vi "Drive Helper.vi"(1 "QuickTurn":bool, 2 "AutoShift":bool, 3 "Wheel Speed":dbl, 5 "Throttle":dbl(slide) scale=-1.0..1.0, 9 "Turn":dbl(slide) scale=-1.0..1.0, 12 "ForceHigh":bool, 13 "ForceLow":bool) -> (6 "Left Output":dbl(slide) scale=-1.0..1.0, 8 "isHighGear":bool, 10 "Right Output":dbl(slide) scale=-1.0..1.0)   [LabVIEW 2014]
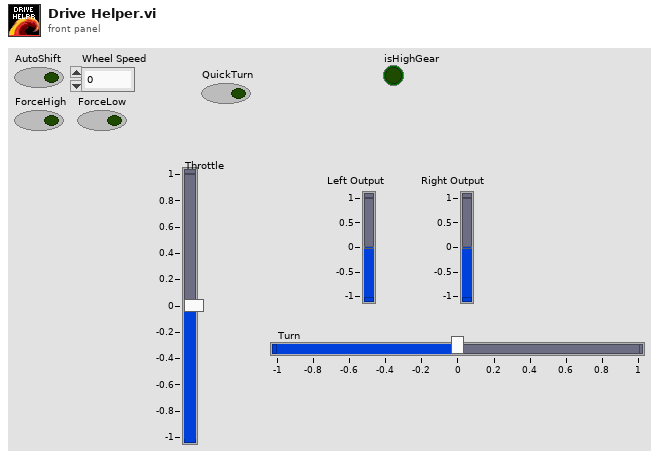
[diagram p1: front panel]
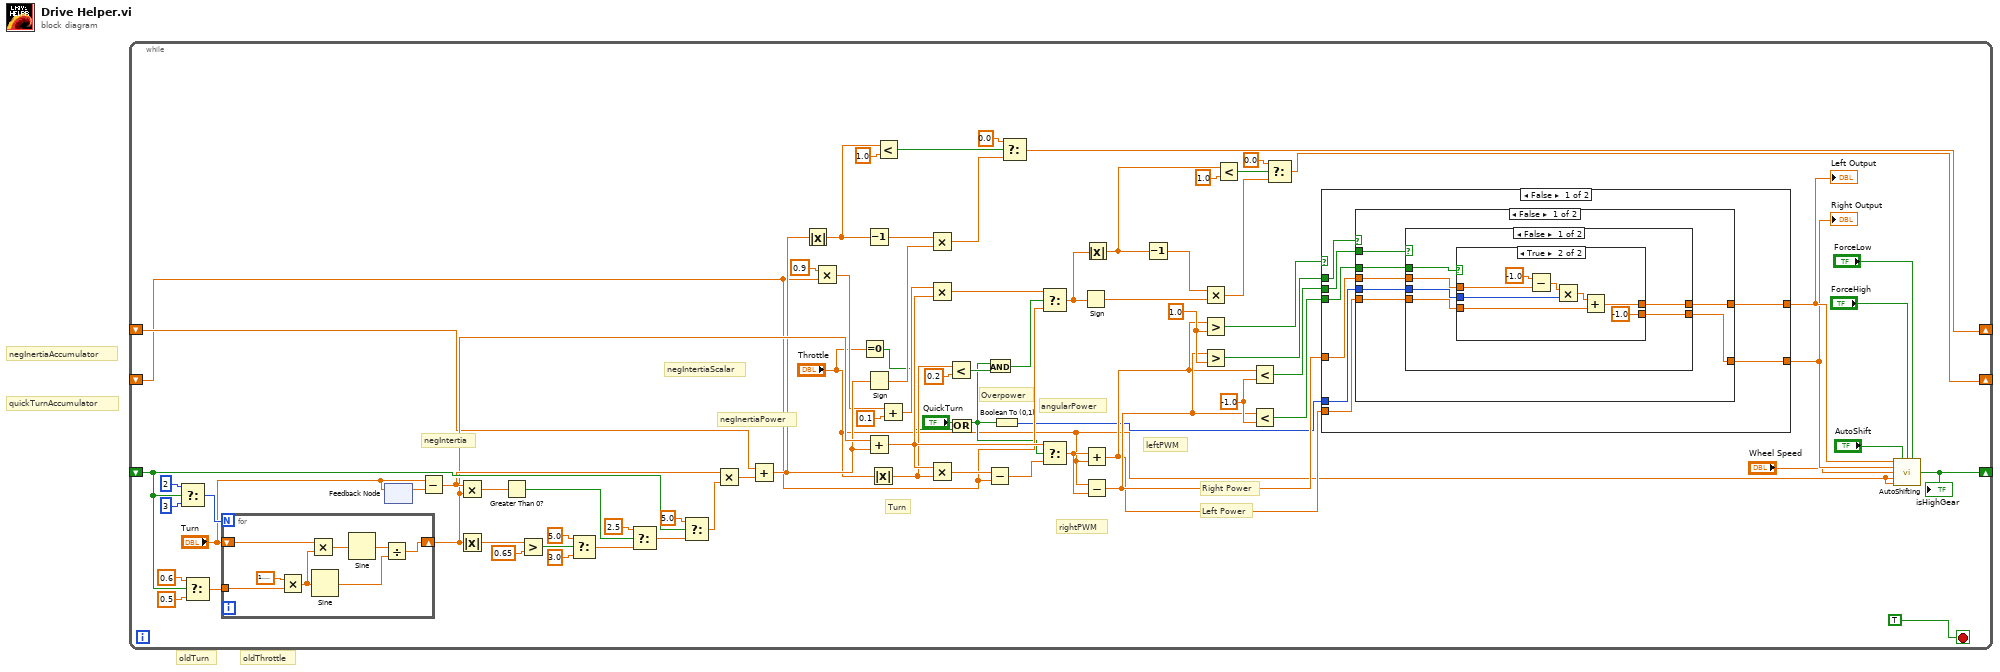
[diagram p0: block diagram]
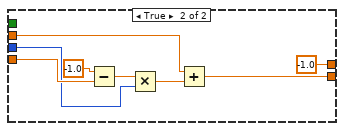
[diagram p3: hidden frame]
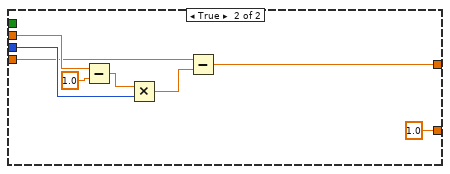
[diagram p4: hidden frame]
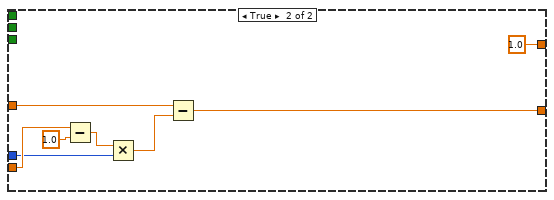
[diagram p5: hidden frame]
diagram:
  # "quickTurnAccumulator"
  # "negInertiaAccumulator"
  # "oldThrottle"
  # "oldTurn"
  n1 = while {
    shift-right: [w77] -> _
    shift-left: _ -> [w69]
    shift-right: [w45] -> _
    shift-left: _ -> [w42]
    shift-right: [w21] -> _
    shift-left: _ -> [w31]
    stop <- TRUE ("Stop") stop-if-true
    w17 = -1.0 ("y")
    w14 = 1.0 ("y")
    # "Right Power"
    # "Left Power"
    # "Overpower"
    # "rightPWM"
    # "leftPWM"
    # "angularPower"
    # "Turn"
    # "negInertiaPower"
    # "negIntertiaScalar"
    # "negIntertia"
    n2 = Select(t=2, s=w69, f=3) -> (s? t:f=w73:i32)
    n3 = Select(t=0.6, s=w69, f=0.5) -> (s? t:f=w76:dbl)
    n4 = for {
      N: w73 -> [_]
      shift-right: [w137] -> w54
      shift-left: "Turn" -> [w134]
      tunnel: w76 -> [w140]
      n5 = Multiply(x=1.5707963267948966, y=w140) -> (x*y=w136:dbl)
      n6 = Multiply(x=w134, y=w136) -> (x*y=w135:dbl)
      n7 = Sine(x=w136) -> (sin(x)=w138:dbl)
      n8 = Sine(x=w135) -> (sin(x)=w139:dbl)
      n9 = Divide(x=w139, y=w138) -> (x/y=w137:dbl)
    }
    n10 = feedback-in #1("Turn") -> ()
    n11 = feedback #1() -> (w70:dbl)  [unwired: 1 in]
    n12 = Subtract(x="Turn", y=w70) -> (x-y=w56:dbl)
    n13 = Multiply(x=w56, y=w54) -> (x*y=w67:dbl)
    n14 = Absolute Value(x=w54) -> (abs(x)=w63:dbl)
    n15 = Greater Than 0?(x=w67) -> (x > 0?=w66:bool)
    n16 = Greater?(x=w63, y=0.65) -> (0:w60:bool)
    n17 = Select(t=5.0, s=w60, f=3.0) -> (s? t:f=w62:dbl)
    n18 = Select(t=2.5, s=w66, f=w62) -> (s? t:f=w61:dbl)
    n19 = Select(t=5.0, s=w69, f=w61) -> (s? t:f=w57:dbl)
    n20 = Multiply(x=w56, y=w57) -> (x*y=w55:dbl)
    n21 = Add(x=w42, y=w55) -> (x+y=w47:dbl)
    n22 = Absolute Value(x=w47) -> (abs(x)=w50:dbl)
    n23 = Multiply(x=0.9, y=w31) -> (x*y=w39:dbl)
    n24 = Equal To 0?(x="Throttle") -> (x = 0?=w1:bool)
    n25 = Decrement(x=w50) -> (x-1=w49:dbl)
    n26 = Sign(1:w47) -> (0:w48:dbl)
    n27 = Add(x=w54, y=w47) -> (x+y=w34:dbl)
    n28 = Absolute Value(x="Throttle") -> (abs(x)=w33:dbl)
    n29 = Less?(x=w50, y=1.0) -> (x < y?=w52:bool)
    n30 = Add(x=w39, y=0.1) -> (x+y=w38:dbl)
    n31 = Multiply(x=w49, y=w48) -> (x*y=w46:dbl)
    n32 = Multiply(x=w38, y=w34) -> (x*y=w37:dbl)
    n33 = Multiply(x=w34, y=w33) -> (x*y=w32:dbl)
    n34 = Less?(x=w33, y=0.2) -> (x < y?=w36:bool)
    n35 = Or(x="QuickTurn", y=w1) -> (x .or. y?=w3:bool)
    n36 = Subtract(x=w32, y=w31) -> (x-y=w30:dbl)
    n37 = And(x=w3, y=w36) -> (x .and. y?=w35:bool)
    n38 = Boolean To (0,1)(Boolean=w3) -> (0, 1=w10:i16)
    n39 = Select(t=0.0, s=w52, f=w46) -> (s? t:f=w45:dbl)
    n40 = Select(t=w37, s=w35, f=w31) -> (s? t:f=w22:dbl)
    n41 = Select(t=w34, s=w3, f=w30) -> (s? t:f=w20:dbl)
    n42 = Sign(1:w22) -> (0:w28:dbl)
    n43 = Add(x=w20, y="Throttle") -> (x+y=w11:dbl)
    n44 = Subtract(x="Throttle", y=w20) -> (x-y=w12:dbl)
    n45 = Absolute Value(x=w22) -> (abs(x)=w26:dbl)
    n46 = Decrement(x=w26) -> (x-1=w27:dbl)
    n47 = Multiply(x=w27, y=w28) -> (x*y=w29:dbl)
    n48 = Greater?(x=w11, y=w14) -> (0:w13:bool)
    n49 = Greater?(x=w12, y=w14) -> (0:w15:bool)
    n50 = Less?(x=w26, y=1.0) -> (x < y?=w24:bool)
    n51 = Less?(x=w11, y=w17) -> (x < y?=w16:bool)
    n52 = Less?(x=w12, y=w17) -> (x < y?=w18:bool)
    n53 = Select(t=0.0, s=w24, f=w29) -> (s? t:f=w21:dbl)
    n54 = case shown="False" w13 {
      tunnel: w15 -> [w86 _]
      tunnel: w16 -> [w85 _]
      tunnel: w18 -> [w84 _]
      tunnel: w11 -> [w80 w133]
      tunnel: w10 -> [w81 w130]
      tunnel: w12 -> [w82 w128]
      tunnel: [w83 w127] -> w6
      tunnel: [w79 1.0] -> w7
      frame False {
        n55 = case shown="False" w86 {
          tunnel: w85 -> [w93 _]
          tunnel: w84 -> [w92 _]
          tunnel: [w88 1.0] -> w83
          tunnel: w82 -> [w89 w121]
          tunnel: w81 -> [w90 w120]
          tunnel: w80 -> [w91 w119]
          tunnel: [w87 w118] -> w79
          frame False {
            n56 = case shown="False" w93 {
              tunnel: w92 -> [w99 _]
              tunnel: w91 -> [w96 w116]
              tunnel: w90 -> [w97 w114]
              tunnel: w89 -> [w98 w112]
              tunnel: [w94 w111] -> w88
              tunnel: [w95 -1.0] -> w87
              frame False {
                n57 = case shown="True" w99 {
                  tunnel: w98 -> [w100 w108]
                  tunnel: w97 -> [_ w106]
                  tunnel: w96 -> [w101 w104]
                  tunnel: [w101 w103] -> w95
                  tunnel: [w100 -1.0] -> w94
                  frame False {
                  }
                  frame True {
                    n58 = Subtract(x=-1.0, y=w108) -> (x-y=w107:dbl)
                    n59 = Multiply(x=w107, y=w106) -> (x*y=w105:dbl)
                    n60 = Add(x=w105, y=w104) -> (x+y=w103:dbl)
                  }
                }
              }
              frame True {
                n61 = Subtract(x=-1.0, y=w116) -> (x-y=w115:dbl)
                n62 = Multiply(x=w115, y=w114) -> (x*y=w113:dbl)
                n63 = Add(x=w112, y=w113) -> (x+y=w111:dbl)
              }
            }
          }
          frame True {
            n64 = Subtract(x=w121, y=1.0) -> (x-y=w124:dbl)
            n65 = Multiply(x=w124, y=w120) -> (x*y=w125:dbl)
            n66 = Subtract(x=w119, y=w125) -> (x-y=w118:dbl)
          }
        }
      }
      frame True {
        n67 = Subtract(x=w133, y=1.0) -> (x-y=w131:dbl)
        n68 = Multiply(x=w131, y=w130) -> (x*y=w129:dbl)
        n69 = Subtract(x=w128, y=w129) -> (x-y=w127:dbl)
      }
    }
    "Left Output" <- w7
    "Right Output" <- w6
    n70 = call "AutoShifting.vi"("LeftPWM"=w7, "AutoShift"="AutoShift", "ForceHigh"="ForceHigh", "ForceLow"="ForceLow", "RightPWM"=w6, "Wheel Speed"="Wheel Speed", "LinearPower"="Throttle", "Throttle"="Throttle") -> ("isHighGear"=w77:bool)  [unwired: 7 in]
    "isHighGear" <- w77
  }
